vi "MVE Search Array With Errors.vi"(9 "String":string, 10 "Array of Strings":string[](array[string]), 11 "error in (no error)":errorcluster) -> (2 "index of element":i32, 3 "error out":errorcluster)   [LabVIEW 2016]
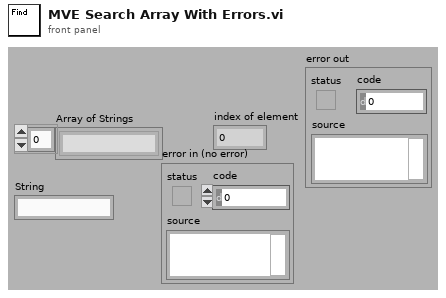
[diagram p1: front panel]
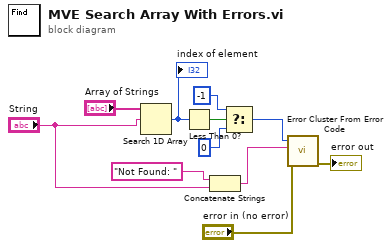
[diagram p0: block diagram]
diagram:
  n1 = Search 1D Array(1D array="Array of Strings", element="String") -> (index of element=w11:i32)  [unwired: 1 in]
  "index of element" <- w11
  n2 = Less Than 0?(x=w11) -> (x < 0?=w9:bool)
  n3 = Concatenate Strings("Not Found: " ("error message (\"\")"), "String") -> (w2:string)
  n4 = Select(t=-1 ("error code (0)"), s=w9, f=0 ("error code (0)")) -> (s? t:f=w6:i32)
  n5 = call <vilib>:"Error Cluster From Error Code.vi"("error in (no error)"="error in (no error)", "error message (\"\")"=w2, "error code (0)"=w6) -> ("error out"=→"error out":errorcluster)  [unwired: 6 in]
